vi "configure.vi"(8 "error in (no error)":errorcluster, 11 "GenericPlugin in":refnum<class "ClockDL100201DAQmx.lvclass">) -> (0 "error out":errorcluster, 3 "GenericPlugin out":refnum<class "ClockDL100201DAQmx.lvclass">)   [LabVIEW 2010, in "ClockDL100201DAQmx.lvclass"]
doc: "The dynamic dispatch version of this VI loads and displays the configuration file associated with the plug-in object. The user modify and save the configuration data."
uses:
  ClockDL100201DAQmx.lvclass
  ClockDL100201DAQmx.lvclass/ClockDL100201DAQmx.ctl
panel:
  in  "period counter":tag
  in  "trigger source":tag
  in  "output terminal":tag
  in  "cancelButton":bool
  in  "saveButton":bool
  # "Configure ClockDL100201DAQmx"
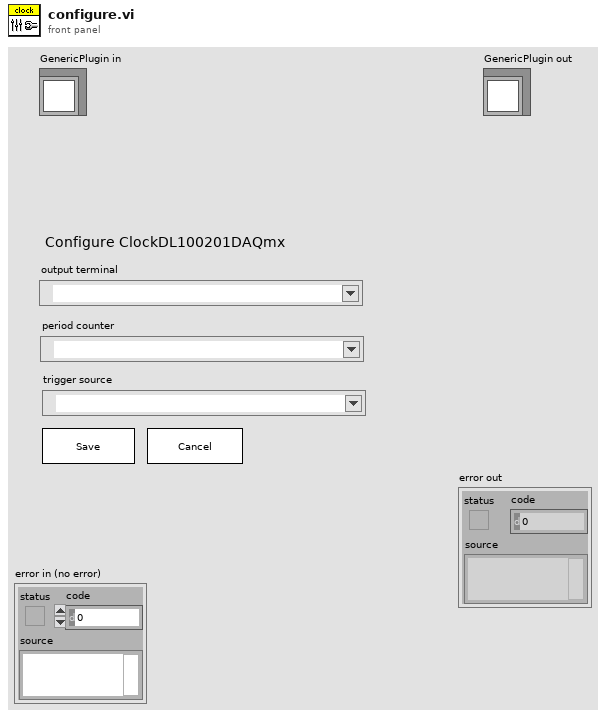
[diagram p1: front panel]
types:
  T1 = typedef "ClockDL100201DAQmx.lvclass/config_data_cluster.ctl" = cluster{"output terminal":string, "trigger source":string, "period counter":string}
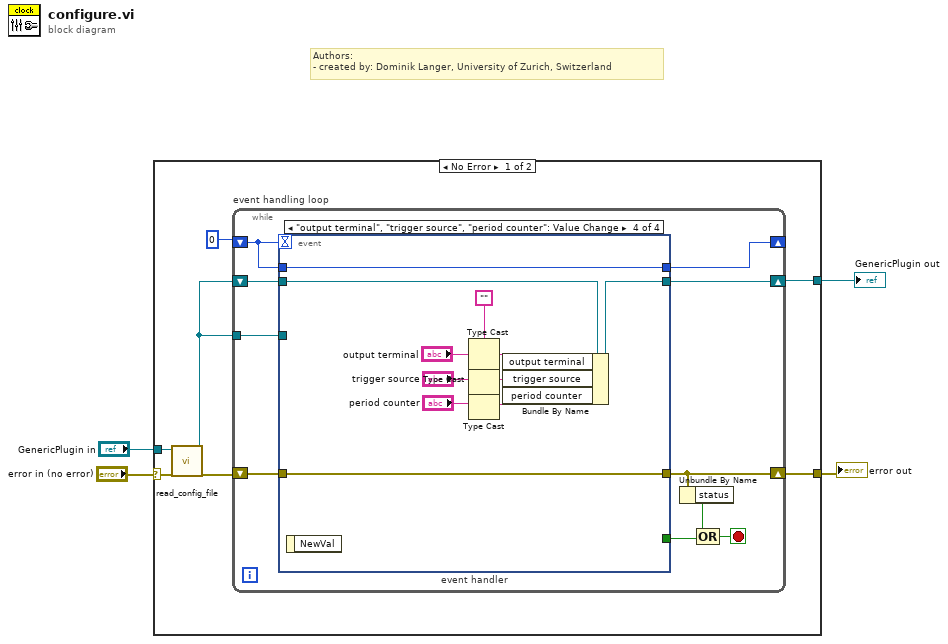
[diagram p0: block diagram]
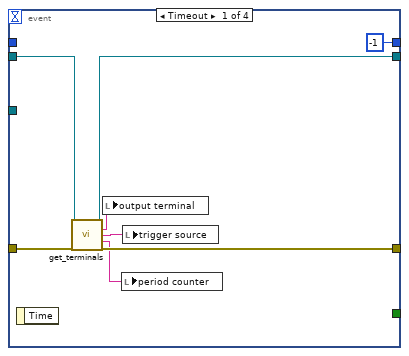
[diagram p2: hidden frame]
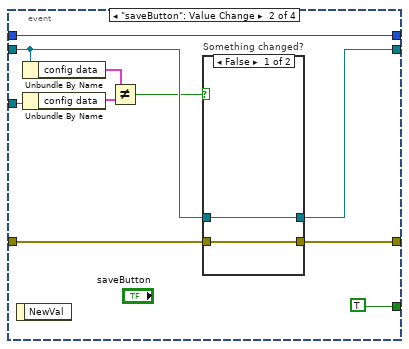
[diagram p3: hidden frame]
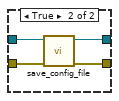
[diagram p4: hidden frame]
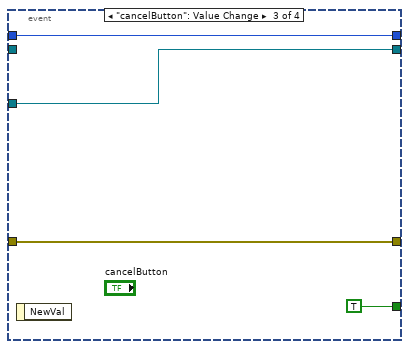
[diagram p5: hidden frame]
diagram:
  # "Authors: \n- created by: Dominik Langer, University of Zurich, Switzerland"
  n1 = case shown="No Error" "error in (no error)" {
    selector: "error in (no error)" -> [w8 w62]
    tunnel: [w10 w62] -> w3
    tunnel: [w9 w61] -> w2
    tunnel: "GenericPlugin in" -> [w6 w61]
    frame No Error {
      n2 = call-dynamic "read_config_file.vi"("error in (no error)"=w8, "GenericPlugin in"=w6) -> ("error out"=w7:errorcluster, "GenericPlugin out"=w5:refnum<class "ClockDL100201DAQmx.lvclass">)  [unwired: 8 in]
      n3 = while "event handling loop" {
        shift-right: [w20] -> _
        shift-left: 0 -> [w21]
        shift-right: [w15] -> w10
        shift-left: w7 -> [w19]
        shift-right: [w17] -> w9
        shift-left: w5 -> [w18]
        tunnel: w5 -> [w16]
        stop <- w12 stop-if-true
        n4 = event "event handler" shown="[3] \"output terminal\", \"trigger source\", \"period counter\": Value Change" {
          selector: _ -> [_ _ _ _]
          dyn-events: _ -> [_ _ _ _]
          timeout: w21 -> [_ _ _ _]
          tunnel: w21 -> [_ w39 w49 w60]
          tunnel: [-1 w39 w49 w60] -> w20
          tunnel: w19 -> [w28 w37 w48 w59]
          tunnel: [w27 w36 w48 w59] -> w15
          tunnel: w18 -> [w26 w34 _ w58]
          tunnel: [w25 w35 w46 w57] -> w17
          tunnel: [_ TRUE TRUE _] -> w14
          tunnel: w16 -> [_ w33 w46 _]
          event Timeout {
            n5 = event-data() -> ()  [unwired: 1 in, 1 out]
            n6 = call-dynamic "get_terminals.vi"("ClockDL100201DAQmx in"=w26, "error in (no error)"=w28) -> ("ClockDL100201DAQmx out"=w25:refnum<class "ClockDL100201DAQmx.lvclass">, "output terminal"=w23:tag, "trigger source"=w24:tag, "period counter"=w22:tag, "error out"=w27:errorcluster)  [unwired: 9 in]
            n7 = local write "output terminal"(w23) -> ()
            n8 = local write "period counter"(w22) -> ()
            n9 = local write "trigger source"(w24) -> ()
          }
          event "saveButton": Value Change {
            n10 = event-data() -> ()  [unwired: 1 in, 1 out]
            n11 = Unbundle By Name(w34) -> ("config data"=w30:T1)
            n12 = Unbundle By Name(w33) -> ("config data"=w32:T1)
            n13 = Not Equal?(x=w30, y=w32) -> (x != y?=w31:bool)
            n14 = case "Something changed?" shown="False" w31 {
              tunnel: w37 -> [w40 w45]
              tunnel: [w40 w44] -> w36
              tunnel: w34 -> [w41 w43]
              tunnel: [w41 w42] -> w35
              frame False {
              }
              frame True {
                n15 = call-dynamic "save_config_file.vi"("error in (no error)"=w45, "GenericPlugin in"=w43) -> ("error out"=w44:errorcluster, "GenericPlugin out"=w42:refnum<class "ClockDL100201DAQmx.lvclass">)  [unwired: 8 in]
              }
            }
          }
          event "cancelButton": Value Change {
            n16 = event-data() -> ()  [unwired: 1 in, 1 out]
          }
          event "output terminal", "trigger source", "period counter": Value Change {
            w52 = ""
            n17 = event-data() -> ()  [unwired: 1 in, 1 out]
            n18 = Type Cast(type=w52, x="output terminal") -> (*(type *) &x=w54:string)
            n19 = Type Cast(type=w52, x="trigger source") -> (*(type *) &x=w55:string)
            n20 = Type Cast(type=w52, x="period counter") -> (*(type *) &x=w50:string)
            n21 = Bundle By Name(cluster=w58, "output terminal"=w54, "trigger source"=w55, "period counter"=w50) -> (w57:refnum<class "ClockDL100201DAQmx.lvclass">)
          }
        }
        n22 = Unbundle By Name(w15) -> ("status"=w13:bool)
        n23 = Compound Arithmetic op=OR(w13, w14) -> (w12:bool)
      }
    }
    frame Error {
    }
  }
  "error out" <- w3
  "GenericPlugin out" <- w2
